vi "Refresh State.vi"(8 "error in":errorcluster, 11 "Base Software in":refnum<class "Base Software.lvclass">) -> (0 "error out":errorcluster, 3 "Base Software out":refnum<class "Base Software.lvclass">)   [LabVIEW 2019, in "Base Software.lvlib" / "Main.lvlib" / "Base Software.lvclass"]
uses:
  Project/Base Software.lvclass
  C:/Users/Public/Documents/Development/builds/Engine/Engine.lvlibp/Project/Engine.lvclass
  Project/Base Software.lvclass/Base Software.ctl
  Custom Controls/Color_Items.ctl
  builds/Engine/Engine.lvlibp/Accessors/Read Self Q.vi
  builds/Engine/Actor Framework.lvlibp/1abvi3w/vi.lib/ActorFramework/Message Enqueuer/Enqueue.vi
  builds/Engine/Actor Framework.lvlibp/1abvi3w/vi.lib/ActorFramework/Message Enqueuer/Message Enqueuer.lvclass
  Base Software Messages/Show Splash Screen Msg/Show Splash Screen Msg.lvclass
  builds/Engine/Engine.lvlibp/Project/Engine.lvclass
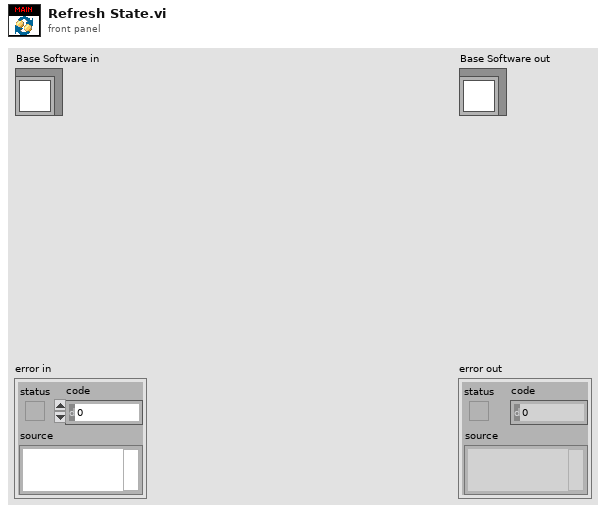
[diagram p1: front panel]
types:
  T1 = typedef "Base Software.lvlib/Main.lvlib/Base Software.lvclass/Color_Items.ctl" = enum16{"Nominal_Low_Impact", "Nominal", "User_Interaction", "Warning", "Error"}
  T2 = typedef "Engine.lvlibp/Engine.lvclass/System Status.ctl" = enum16{"Logged Off", "UUT_Info_Missing", "Idle", "Error", "Warning", "Loading", "Config", "Manual", "Automation", "Report_View", "Previous"}
  T3 = typedef "LVTextColorsTypeDef.ctl" = cluster{"Text Color":u32, "Background Color":u32}
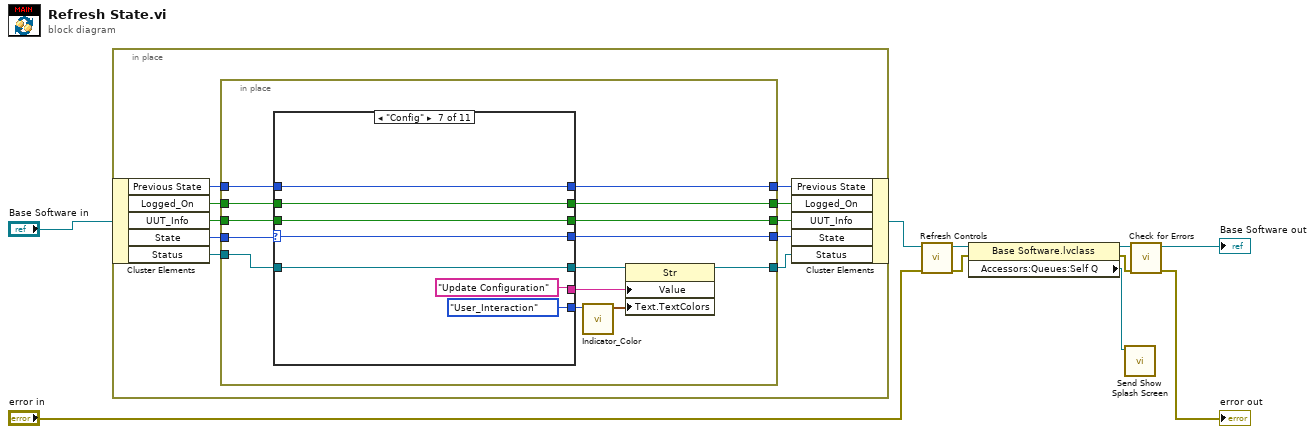
[diagram p0: block diagram]
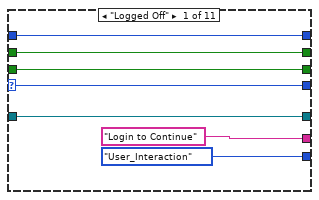
[diagram p2: hidden frame]
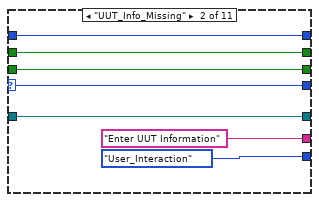
[diagram p3: hidden frame]
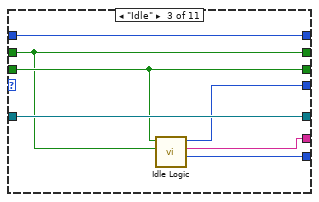
[diagram p4: hidden frame]
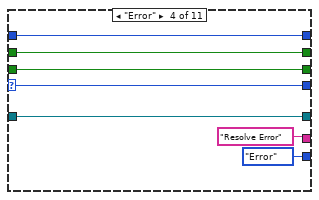
[diagram p5: hidden frame]
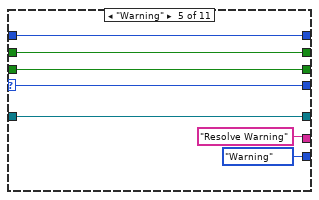
[diagram p6: hidden frame]
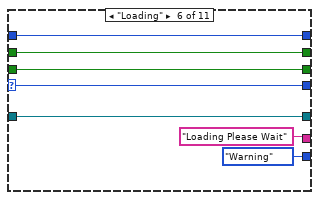
[diagram p7: hidden frame]
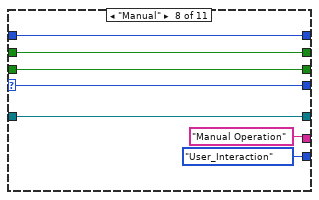
[diagram p8: hidden frame]
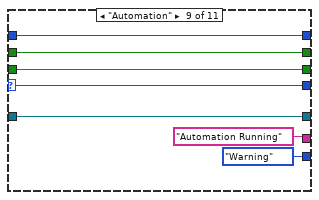
[diagram p9: hidden frame]
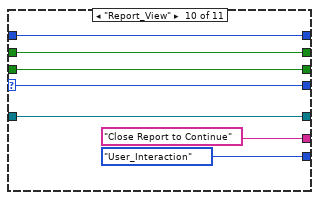
[diagram p10: hidden frame]
diagram:
  n1 = in-place {
    n2 = in-place-cluster #1("Base Software in") -> ("Previous State"=w14:T2, "Logged_On"=w18:bool, "UUT_Info"=w17:bool, "State"=w20:T2, "Status"=w12:refnum<vi>)
    n3 = in-place {
      in-place-border: w20 -> [w34]
      in-place-border: [w33] -> w19
      in-place-border: w18 -> [w28]
      in-place-border: w17 -> [w27]
      in-place-border: [w26] -> w16
      in-place-border: [w25] -> w15
      in-place-border: w14 -> [w24]
      in-place-border: [w23] -> w13
      in-place-border: w12 -> [w22]
      in-place-border: [w21] -> w11
      n4 = case shown="\"Config\"" w34 {
        selector: w34 -> [w41 w48 _ w61 w68 w75 w82 w89 w96 w104 _]
        tunnel: w22 -> [w40 w47 w55 w62 w69 w76 w83 w90 w97 w103 w106]
        tunnel: [w40 w47 w55 w62 w69 w76 w83 w90 w97 w103 w106] -> w32
        tunnel: [w41 w48 w50 w61 w68 w75 w82 w89 w96 w104 w105] -> w33
        tunnel: [Color_Items."User_Interaction" ("Color Selector") Color_Items."User_Interaction" ("Color Selector") w52 Color_Items."Error" ("Color Selector") Color_Items."Warning" ("Color Selector") Color_Items."Warning" ("Color Selector") Color_Items."User_Interaction" ("Color Selector") Color_Items."User_Interaction" ("Color Selector") Color_Items."Warning" ("Color Selector") Color_Items."User_Interaction" ("Color Selector") _] -> w30
        tunnel: ["Login to Continue" "Enter UUT Information" w51 "Resolve Error" "Resolve Warning" "Loading Please Wait" "Update Configuration" "Manual Operation" "Automation Running" "Close Report to Continue" _] -> w29
        tunnel: w28 -> [w37 w44 w53 w58 w65 w72 w79 w86 w93 w100 w108]
        tunnel: w27 -> [w36 w43 w54 w57 w64 w71 w78 w85 w92 w99 w107]
        tunnel: [w37 w44 w53 w58 w65 w72 w79 w86 w93 w100 w108] -> w26
        tunnel: [w36 w43 w54 w57 w64 w71 w78 w85 w92 w99 w107] -> w25
        tunnel: w24 -> [w35 w42 w49 w56 w63 w70 w77 w84 w91 w98 w105]
        tunnel: [w35 w42 w49 w56 w63 w70 w77 w84 w91 w98 w105] -> w23
        frame "Logged Off" {
        }
        frame "UUT_Info_Missing" {
        }
        frame "Idle" {
          n5 = call "Idle Logic.vi"("Logged on"=w53, "UUT Info"=w54) -> ("Color Selector"=w52:T1, "String"=w51:string, "State"=w50:T2)  [unwired: 7 in]
        }
        frame "Error" {
        }
        frame "Warning" {
        }
        frame "Loading" {
        }
        frame "Config" {
        }
        frame "Manual" {
        }
        frame "Automation" {
        }
        frame "Report_View" {
        }
        frame "Previous" {
        }
      }
      n6 = call "Indicator_Color.vi"("Color Selector"=w30) -> ("Text Colors"=w31:T3)  [unwired: 10 in]
      n7 = property class="Str"(reference=w32, "Value"=w29, "Text.TextColors"=w31) -> (reference out=w21:refnum<vi>)  [unwired: 1 in, 1 out]
    }
    n8 = in-place-cluster #1("Previous State"=w13, "Logged_On"=w16, "UUT_Info"=w15, "State"=w19, "Status"=w11) -> (w7:refnum<class "Base Software.lvclass">)
  }
  n9 = call "Refresh Controls.vi"("error in"="error in", "Base Software in"=w7) -> ("error out"=w4:errorcluster, "Base Software out"=w5:refnum<class "Base Software.lvclass">)  [unwired: 8 in]
  n10 = property class="Base Software.lvclass"(reference=w5, error in=w4) -> (reference out=w2:refnum<class "Base Software.lvclass">, error out=w1:errorcluster, "Accessors:Queues:Self Q"=w3:refnum<class "Message Enqueuer.lvclass">)
  n11 = call "Send Show Splash Screen.vi"("Message Enqueuer"=w3) -> ()  [unwired: 9 in, 2 out]
  n12 = call "Check for Errors.vi"("error in"=w1, "Engine in"=w2) -> ("error out"=→"error out":errorcluster, "Engine out"=→"Base Software out":refnum<class "Base Software.lvclass">)  [unwired: 8 in]
